vi "getPayloadRequirement.vi"(11 "PUBLISH in":refnum<class "PUBLISH.lvclass">) -> (2 "Requirement":T1, 3 "PUBLISH out":refnum<class "PUBLISH.lvclass">)   [LabVIEW 2013, in "PUBLISH.lvclass"]
uses:
  PUBLISH.lvclass
  Requirement -- enum.ctl
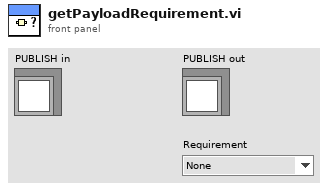
[diagram p1: front panel]
types:
  T1 = typedef "Requirement -- enum.ctl" = enum16{"None", "Optional", "Required"}
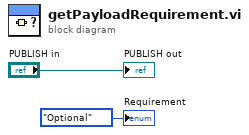
[diagram p0: block diagram]
diagram:
  "PUBLISH out" <- "PUBLISH in"
  "Requirement" <- Requirement_--_enum."Optional" ("Requirement")
